vi "Initialize Configuration Resource.vi"(8 "error in (no error)":errorcluster, 11 "IniFileSection in":refnum<class "IniFileSection.lvclass">) -> (0 "error out":errorcluster, 3 "IniFileSection out":refnum<class "IniFileSection.lvclass">)   [LabVIEW 2017, in "IniFileSection.lvclass"]
uses:
  IniFileSection.lvclass
  IniFileSection.lvclass/IniFileSection.ctl
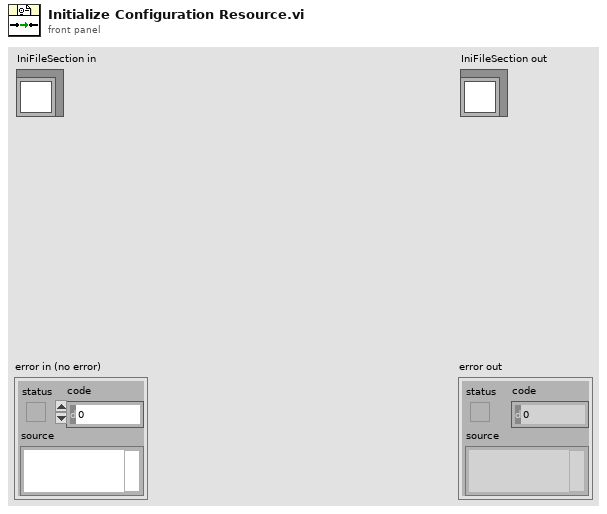
[diagram p1: front panel]
types:
  T1 = enum16{"open", "replace", "create", "open or create", "replace or create", "replace or create with confirmation"}
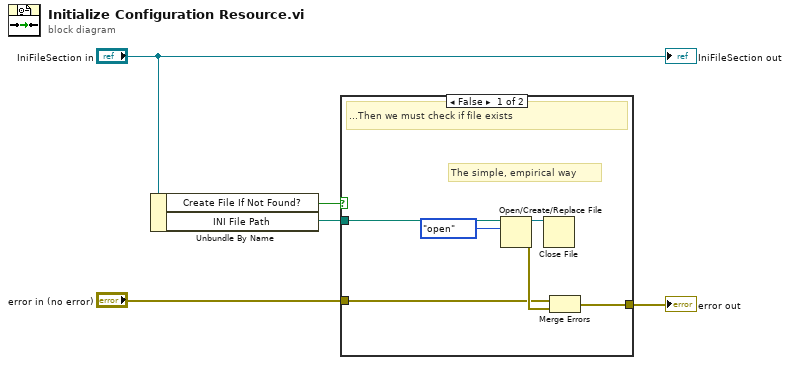
[diagram p0: block diagram]
diagram:
  n1 = Unbundle By Name("IniFileSection in") -> ("Create File If Not Found?"=w1:bool, "INI File Path"=w2:path)
  n2 = case shown="False" w1 {
    tunnel: "error in (no error)" -> [w7 w12]
    tunnel: [w8 w12] -> w3
    tunnel: w2 -> [w6 _]
    frame False {
      # "The simple, empirical way"
      # "...Then we must check if file exists"
      n3 = Open/Create/Replace File(file path (use dialog)=w6, operation (0:open)=T1."open") -> (refnum out=w9:refnum<file>, error out=w11:errorcluster)  [unwired: 4 in, 1 out]
      n4 = Close File(refnum=w9) -> ()  [unwired: 1 in, 2 out]
      n5 = Merge Errors(w7, w11) -> (w8:errorcluster)
    }
    frame True {
      # "No need to check for file"
    }
  }
  "error out" <- w3
  "IniFileSection out" <- "IniFileSection in"
